vi "set_config_cluster.vi"(8 "error in (no error)":errorcluster, 10 "config cluster variant":variant, 11 "DataCollectionMG091001IntrinsicImaging in":refnum<class "DataCollectionMG091001IntrinsicImaging.lvclass">) -> (0 "error out":errorcluster, 3 "DataCollectionMG091001IntrinsicImaging out":refnum<class "DataCollectionMG091001IntrinsicImaging.lvclass">)   [LabVIEW 2010, in "DataCollectionMG091001IntrinsicImaging.lvclass"]
uses:
  DataCollectionMG091001IntrinsicImaging.lvclass
  DataCollectionMG091001IntrinsicImaging.lvclass/DataCollectionMG091001IntrinsicImaging.ctl
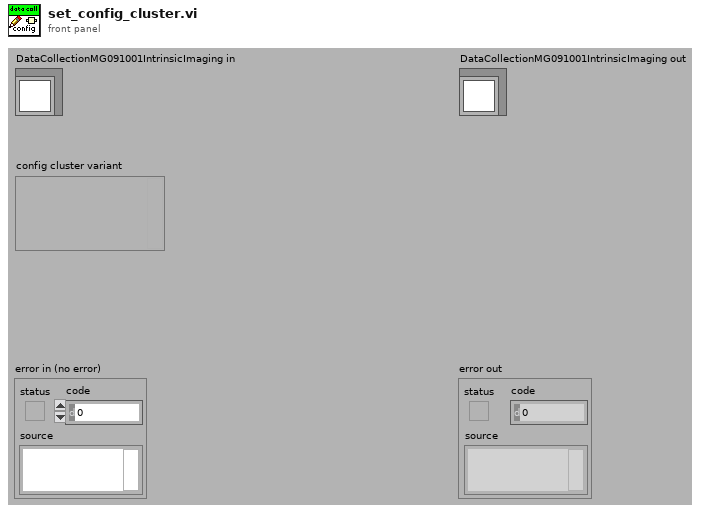
[diagram p1: front panel]
types:
  T1 = typedef "DataCollectionMG091001IntrinsicImaging.lvclass/config_data_cluster.ctl" = cluster{"image multiplication factor":dbl}
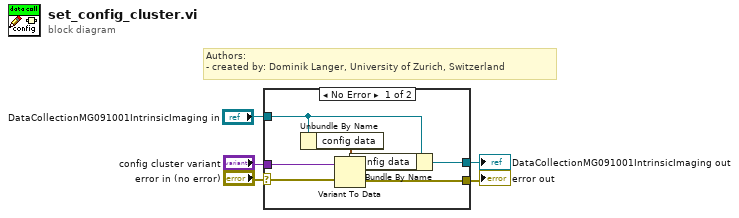
[diagram p0: block diagram]
diagram:
  # "Authors: \n- created by: Dominik Langer, University of Zurich, Switzerland"
  n1 = case shown="No Error" "error in (no error)" {
    selector: "error in (no error)" -> [w12 w13]
    tunnel: [w11 w13] -> w1
    tunnel: "DataCollectionMG091001IntrinsicImaging in" -> [w7 w14]
    tunnel: "config cluster variant" -> [w9 _]
    tunnel: [w6 w14] -> w2
    frame No Error {
      n2 = Unbundle By Name(w7) -> ("config data"=w10:T1)
      n3 = Variant To Data(error in=w12, Variant=w9, type=w10) -> (error out=w11:errorcluster, data=w8:T1)
      n4 = Bundle By Name(cluster=w7, "config data"=w8) -> (w6:refnum<class "DataCollectionMG091001IntrinsicImaging.lvclass">)
    }
    frame Error {
    }
  }
  "error out" <- w1
  "DataCollectionMG091001IntrinsicImaging out" <- w2
